vi "Wait for Start.vi"(8 "error in (no error)":errorcluster, 11 "Game Engine in":refnum<class "Game Engine.lvclass">) -> (0 "error out":errorcluster, 3 "Game Engine out":refnum<class "Game Engine.lvclass">)   [LabVIEW 2017, in "Game Engine.lvlib" / "Game Engine.lvclass"]
uses:
  Game Engine.lvclass
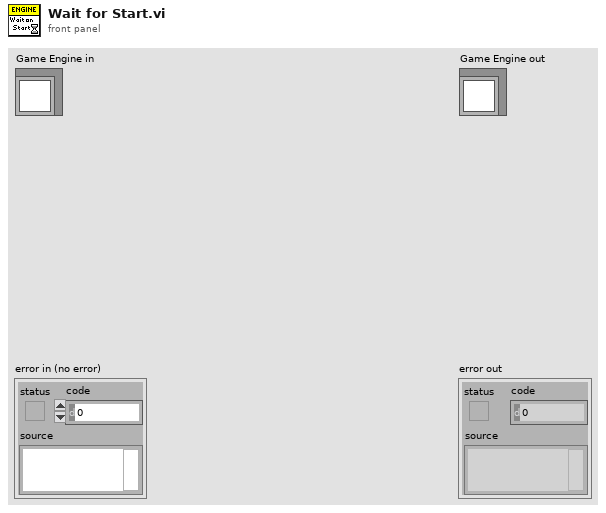
[diagram p1: front panel]
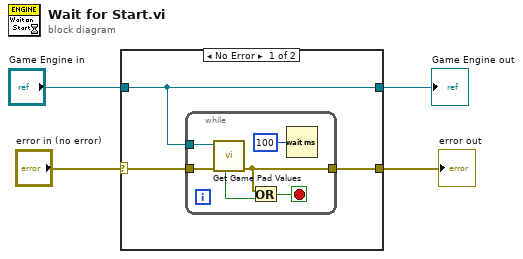
[diagram p0: block diagram]
diagram:
  n1 = case shown="No Error" "error in (no error)" {
    selector: "error in (no error)" -> [w6 w15]
    tunnel: [w5 w15] -> w3
    tunnel: [w7 w14] -> w1
    tunnel: "Game Engine in" -> [w7 w14]
    frame No Error {
      n2 = while {
        tunnel: w7 -> [w13]
        tunnel: w6 -> [w11]
        tunnel: [w8] -> w5
        stop <- w10 stop-if-true
        n3 = call "Get Game Pad Values.vi"("error in (no error)"=w11, "Game Engine in"=w13) -> ("error out"=w8:errorcluster, "Start"=w9:bool)  [unwired: 3 in, 5 out]
        n4 = Or(x=w8, y=w9) -> (x .or. y?=w10:bool)
        n5 = Wait (ms)(milliseconds to wait=u32 100) -> ()  [unwired: 1 out]
      }
    }
    frame Error {
    }
  }
  "error out" <- w3
  "Game Engine out" <- w1
